vi "Write connect.vi"(8 "error in (no error)":errorcluster, 10 "connect":bool, 11 "Y_H in":refnum<class "Y_H.lvclass">) -> (0 "error out":errorcluster, 3 "Y_H out":refnum<class "Y_H.lvclass">)   [LabVIEW 2019, in "Y_H.lvclass"]
uses:
  Y_H.lvclass
  Y_H.lvclass/Y_H.ctl
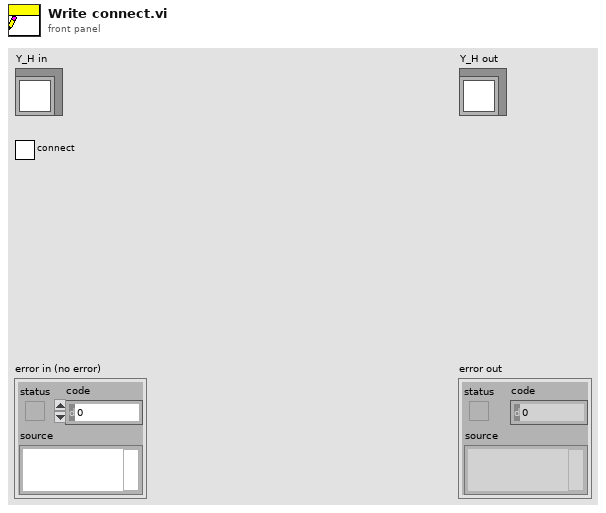
[diagram p1: front panel]
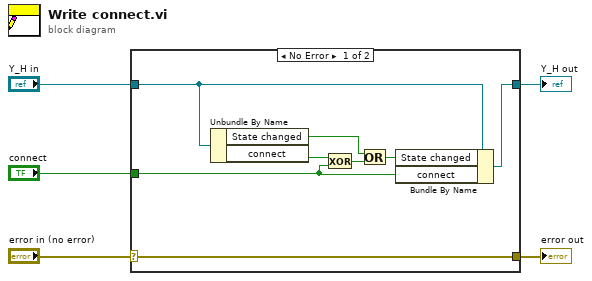
[diagram p0: block diagram]
diagram:
  n1 = case shown="No Error" "error in (no error)" {
    selector: "error in (no error)" -> [w13 w14]
    tunnel: [w13 w14] -> w4
    tunnel: [w12 w15] -> w2
    tunnel: "Y_H in" -> [w11 w15]
    tunnel: "connect" -> [w9 _]
    frame No Error {
      n2 = Unbundle By Name(w11) -> ("State changed"=w6:bool, "connect"=w10:bool)
      n3 = Exclusive Or(1:w9, 2:w10) -> (0:w8:bool)
      n4 = Or(x=w6, y=w8) -> (x .or. y?=w7:bool)
      n5 = Bundle By Name(cluster=w11, "State changed"=w7, "connect"=w9) -> (w12:refnum<class "Y_H.lvclass">)
    }
    frame Error {
    }
  }
  "error out" <- w4
  "Y_H out" <- w2
